vi "getStatusBits.vi"(8 "error in (no error)":errorcluster, 11 "Axis in":refnum<class "Axis.lvclass">) -> (0 "error out":errorcluster, 2 "StatusBits":T1, 3 "Axis out":refnum<class "Axis.lvclass">)   [LabVIEW 2019, in "Axis.lvclass"]
uses:
  Axis.lvclass
  Axis.lvclass/Axis.ctl
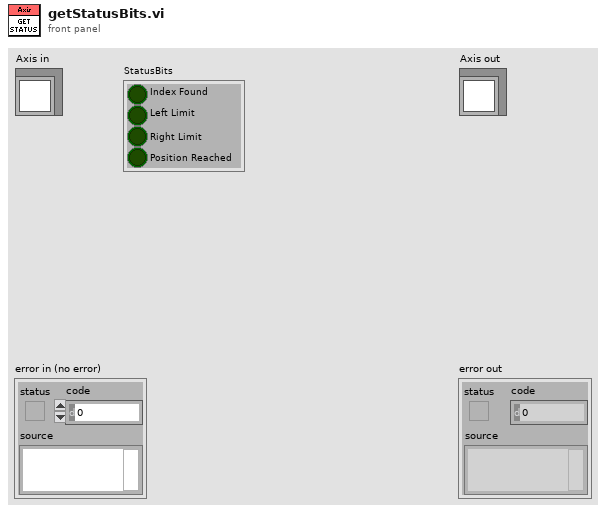
[diagram p1: front panel]
types:
  T1 = cluster{"Index Found":bool, "Left Limit":bool, "Right Limit":bool, "Position Reached":bool}
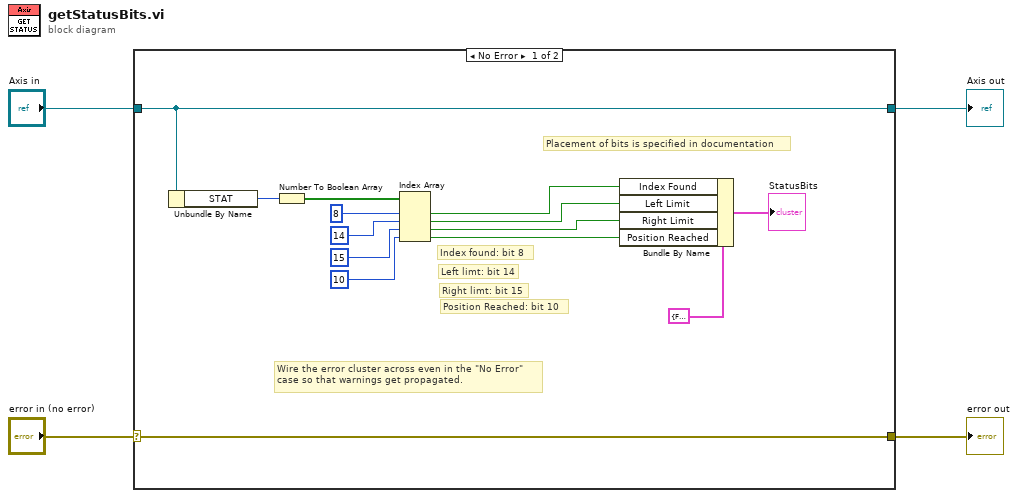
[diagram p0: block diagram]
diagram:
  n1 = case shown="No Error" "error in (no error)" {
    selector: "error in (no error)" -> [w18 w20]
    tunnel: [w18 w20] -> w3
    tunnel: [w15 w19] -> w1
    tunnel: "Axis in" -> [w15 w19]
    frame No Error {
      # "Position Reached: bit 10"
      # "Right limt: bit 15"
      # "Left limt: bit 14"
      # "Index found: bit 8"
      # "Placement of bits is specified in documentation"
      # "Wire the error cluster across even in the \"No Error\"\ncase so that warnings get propagated."
      n2 = Unbundle By Name(w15) -> ("STAT"=w17:i32)
      n3 = Number To Boolean Array(number=w17) -> (Boolean array=w9:bool[])
      n4 = Index Array(array=w9, index #1=8 ("index"), index #2=14 ("index"), index #3=15 ("index"), index #4=10 ("index")) -> (element #1=w8:bool, element #2=w5:bool, element #3=w7:bool, element #4=w6:bool)
      n5 = Bundle By Name(cluster=T1 {"Index Found"=FALSE, "Left Limit"=FALSE, "Right Limit"=FALSE, "Position Reached"=FALSE} ("StatusBits"), "Index Found"=w8, "Left Limit"=w5, "Right Limit"=w7, "Position Reached"=w6) -> (→"StatusBits":T1)
    }
    frame Error {
    }
  }
  "error out" <- w3
  "Axis out" <- w1
